vi "double slider.vi"() -> ()   [LabVIEW 2020]
panel:
  out "String":string
  in  "Horizontal Pointer Slide":cluster{"Numeric":dbl, "Numeric":dbl}(slide) scale=0.0..1920.0
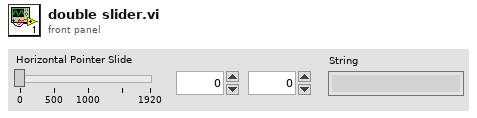
[diagram p1: front panel]
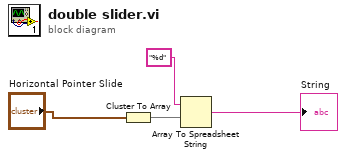
[diagram p0: block diagram]
diagram:
  n1 = Cluster To Array(cluster="Horizontal Pointer Slide") -> (array=w3:dbl[])
  n2 = Array To Spreadsheet String(array=w3, 3:"%d") -> (spreadsheet string=→"String":string)  [unwired: 1 in]
